vi "Set QDList.vi"(8 "error in (no error)":errorcluster, 10 "QDDialogList":refnum<class "QDDialogList.lvclass">, 11 "ScriptSetting in":refnum<class "ScriptSetting.lvclass">) -> (0 "error out":errorcluster, 3 "ScriptSetting out":refnum<class "ScriptSetting.lvclass">)   [LabVIEW 2015, in "ScriptSetting.lvclass"]
uses:
  ScriptSetting.lvclass
  QDSearchList/QDDialogList.lvclass
  ScriptSetting.lvclass/ScriptSetting.ctl
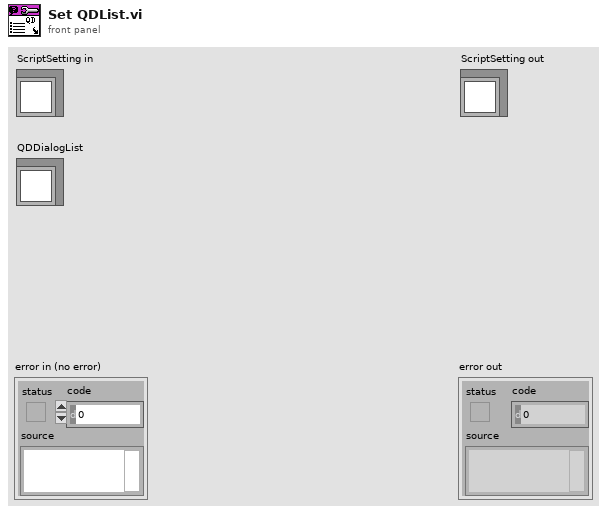
[diagram p1: front panel]
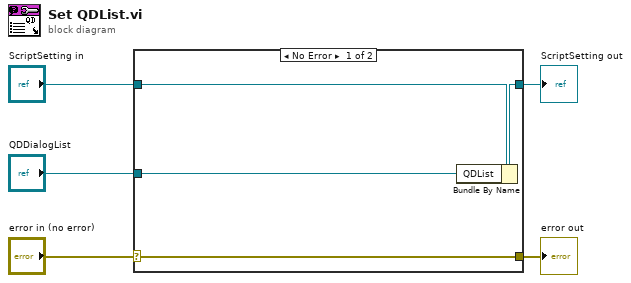
[diagram p0: block diagram]
diagram:
  n1 = case shown="No Error" "error in (no error)" {
    selector: "error in (no error)" -> [w9 w10]
    tunnel: [w9 w10] -> w4
    tunnel: [w7 w11] -> w2
    tunnel: "ScriptSetting in" -> [w8 w11]
    tunnel: "QDDialogList" -> [w6 _]
    frame No Error {
      n2 = Bundle By Name(cluster=w8, "QDList"=w6) -> (w7:refnum<class "ScriptSetting.lvclass">)
    }
    frame Error {
    }
  }
  "error out" <- w4
  "ScriptSetting out" <- w2
